vi "Write Instrument Base.vi"(8 "error in (no error)":errorcluster, 10 "HAL GOOP4.lvlib:Instrument Base":refnum<class "Instr Base.lvclass">, 11 "Virt Instrument Base in":refnum<class "Virt Instr Base.lvclass">) -> (0 "error out":errorcluster, 3 "Virt Instrument Base out":refnum<class "Virt Instr Base.lvclass">)   [LabVIEW 2023, in "HAL GOOP4.lvlib" / "Virt Instr Base.lvclass"]
uses:
  Virt Instr Base.lvclass
  Instrument Base/Instr Base.lvclass
  Virt Instr Base.lvclass/Virt Instr Base.ctl
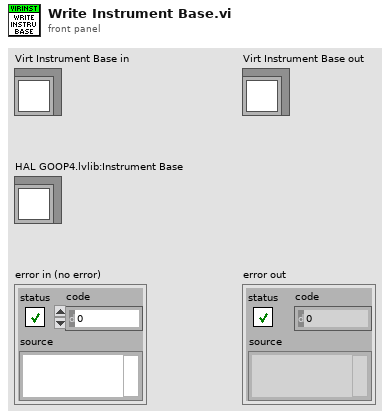
[diagram p1: front panel]
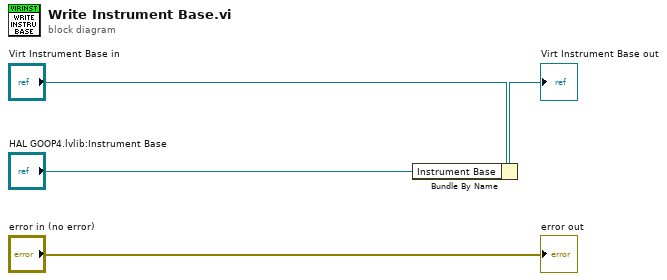
[diagram p0: block diagram]
diagram:
  n1 = Bundle By Name(cluster="Virt Instrument Base in", "Instrument Base"="HAL GOOP4.lvlib:Instrument Base") -> (→"Virt Instrument Base out":refnum<class "Virt Instr Base.lvclass">)
  "error out" <- "error in (no error)"
